vi "cw_5_3b.vi"() -> ()   [LabVIEW 2022 SP3]
panel:
  out "Array":bool[][](array[boolean])
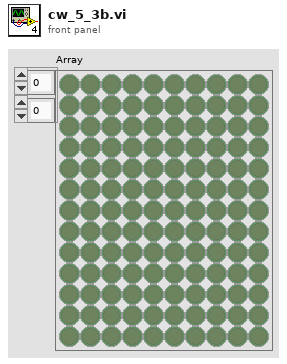
[diagram p1: front panel]
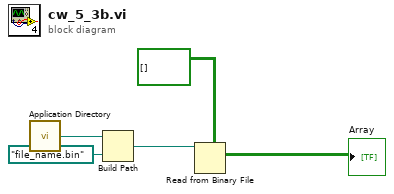
[diagram p0: block diagram]
diagram:
  n1 = call <vilib>:"Application Directory.vi"() -> ("Application Directory"=w5:path)
  n2 = Build Path(base path=w5, name or relative path=path "file_name.bin") -> (appended path=w3:path)
  n3 = Read from Binary File(5:bool[][] [], 11:w3) -> (2:→"Array":bool[][])  [unwired: 4 in, 3 out]
